vi "写入Allowed VI Path.vi"(8 "error in (no error)":errorcluster caption="错误输入（无错误）", 10 "Allowed VI Path":path[](array[path]), 11 "PanelDataNode输入":refnum<class "PanelDataNode.lvclass">) -> (0 "error out":errorcluster caption="错误输出", 3 "PanelDataNode输出":refnum<class "PanelDataNode.lvclass">)   [LabVIEW 2013, in "PanelDataNode.lvclass"]
uses:
  PanelDataNode.lvclass
  PanelDataNode.lvclass/PanelDataNode.ctl
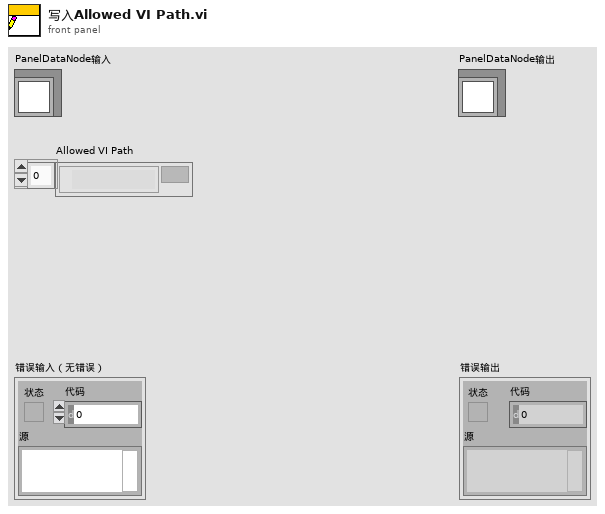
[diagram p1: front panel]
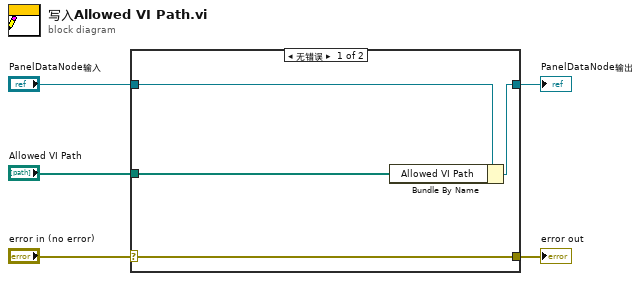
[diagram p0: block diagram]
diagram:
  n1 = case shown="无错误" "error in (no error)" {
    selector: "error in (no error)" -> [w9 w10]
    tunnel: [w9 w10] -> w4
    tunnel: [w7 w11] -> w2
    tunnel: "PanelDataNode输入" -> [w8 w11]
    tunnel: "Allowed VI Path" -> [w6 _]
    frame No Error {
      n2 = Bundle By Name(cluster=w8, "Allowed VI Path"=w6) -> (w7:refnum<class "PanelDataNode.lvclass">)
    }
    frame Error {
    }
  }
  "error out" <- w4
  "PanelDataNode输出" <- w2
